vi "Test_FormatType_CustomCluster_IncludeAllContentsvi.vi"(8 "error in (no error)":errorcluster, 11 "TestCase in":refnum<class "TestVariantExtensions.lvclass">) -> (0 "error out":errorcluster, 3 "TestCase out":refnum<class "TestVariantExtensions.lvclass">)   [LabVIEW 2017, in "TestVariantExtensions.lvclass"]
uses:
  TestVariantExtensions.lvclass
  Source/VariantExtensions.lvlib
panel:
  out "Type String":string
  out "Returned Error (None)":errorcluster
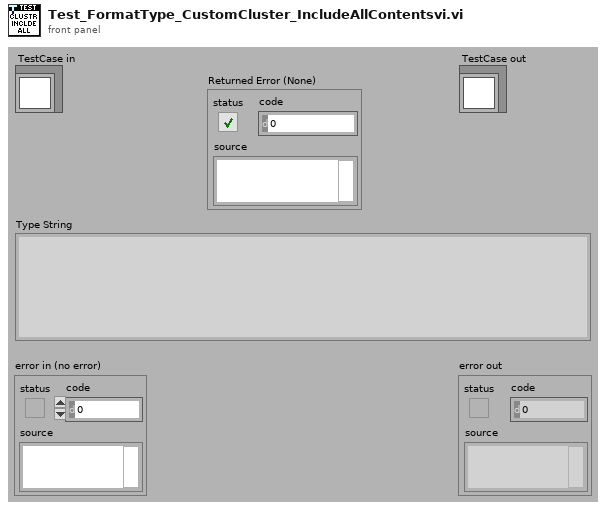
[diagram p1: front panel]
types:
  T1 = cluster{bool, variant, cluster{dbl, u8, string, cluster{timestamp, i32, cluster{path}}[]}}
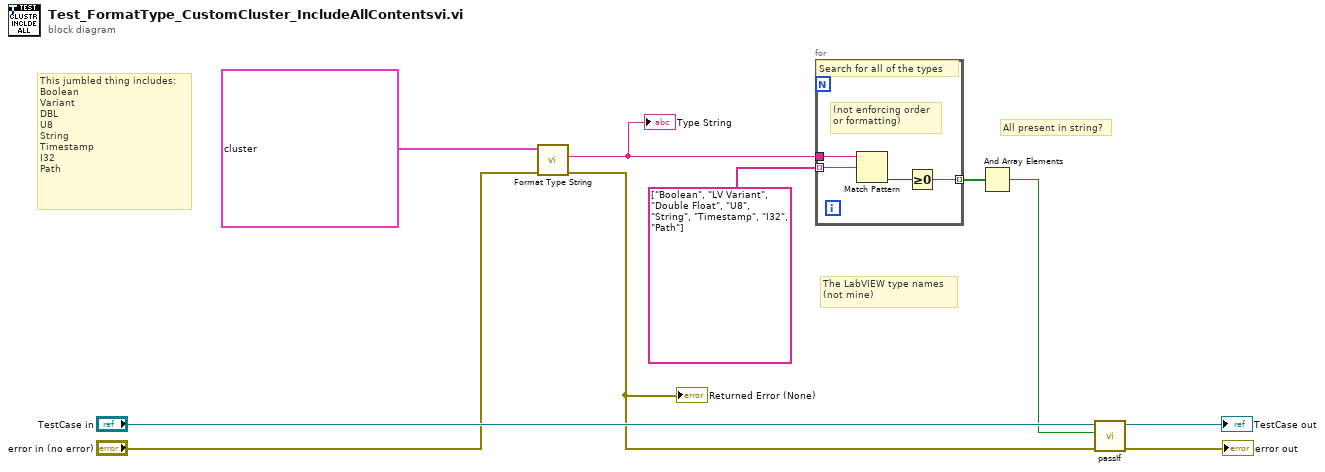
[diagram p0: block diagram]
diagram:
  # "The LabVIEW type names\n(not mine)"
  # "All present in string?"
  # "This jumbled thing includes:\nBoolean\nVariant\nDBL\nU8\nString\nTimestamp\nI32\nPath"
  n1 = call "Format Type String.vi"("error in (no error)"="error in (no error)", "Data Type"=T1 {FALSE, variant, {0.0, 0, "", []}}) -> ("error out"=w6:errorcluster, "Type Name"=w4:string)  [unwired: 8 in]
  "Returned Error (None)" <- w6
  "Type String" <- w4
  n2 = for {
    tunnel: w4 -> [w14]
    tunnel: string[] ["Boolean", "LV Variant", "Double Float", "U8", "String", "Timestamp", "I32", "Path"] ("regular expression") -> [w13] mode=indexing
    tunnel: [w11] -> w2 mode=indexing
    # "(not enforcing order\nor formatting)"
    # "Search for all of the types"
    n3 = Match Pattern(string=w14, regular expression=w13) -> (offset past match=w12:i32)  [unwired: 1 in, 3 out]
    n4 = Greater Or Equal To 0?(x=w12) -> (x >= 0?=w11:bool)
  }
  n5 = And Array Elements(Boolean array=w2) -> (logical AND=w1:bool)
  n6 = call-dynamic "passIf.vi"("error in (no error)"=w6, "pass"=w1, "TestCase in"="TestCase in") -> ("error out"=→"error out":errorcluster, "TestCase out"=→"TestCase out":refnum<class "TestVariantExtensions.lvclass">)  [unwired: 7 in]
